vi "Element to Enum Metadata.vi"(8 "error in (no error)":errorcluster, 9 "Name":string, 10 "MessageElementType":T2, 11 "Element":variant) -> (0 "error out":errorcluster, 2 "Is Enum?":bool, 3 "Enum Metadata":T1)   [LabVIEW 2019, in "grpc-lvsupport.lvlib"]
uses:
  grpc-lvsupport.lvlib
  typeDefs/Message Element Type.ctl
  typeDefs/Enum Metadata.ctl
  <vilib>/Utility/Data Type/NI_Data Type.lvlib
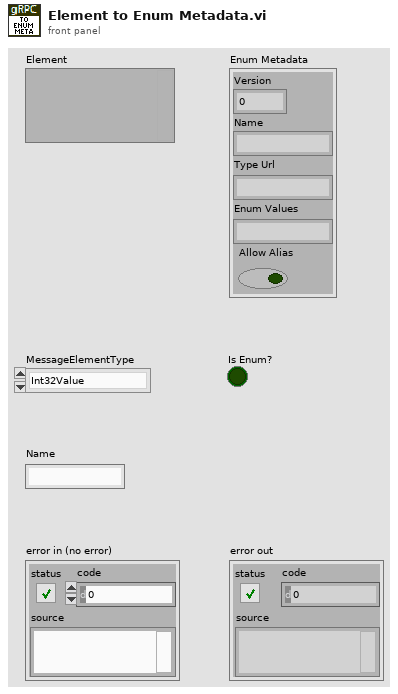
[diagram p1: front panel]
types:
  T1 = typedef "grpc-lvsupport.lvlib/Enum Metadata.ctl" = cluster{"Version":i32, "Name":string, "Type Url":string, "Enum Values":string, "Allow Alias":bool}
  T2 = typedef "grpc-lvsupport.lvlib/Message Element Type.ctl" = enum32{"Int32Value", "FloatValue", "DoubleValue", "BoolValue", "StringValue", "MessageValue", "Int64Value", "UInt32Value", "UInt64Value", "EnumValue", "Bytes", "Fixed64", "Fixed32", "SFixed64", "SFixed32", "SInt64", "SInt32"}
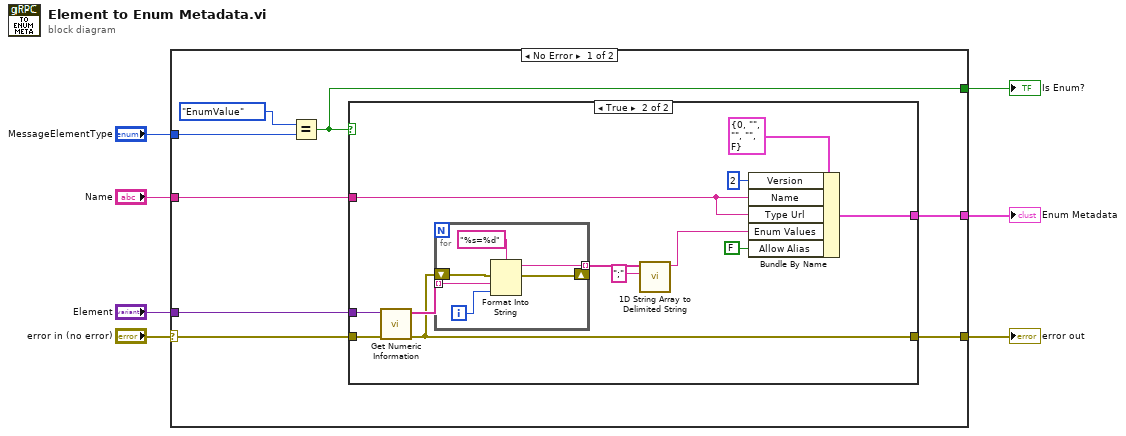
[diagram p0: block diagram]
diagram:
  n1 = case shown="No Error" "error in (no error)" {
    selector: "error in (no error)" -> [w11 w35]
    tunnel: "MessageElementType" -> [w15 _]
    tunnel: [w13 w35] -> w5
    tunnel: "Element" -> [w12 _]
    tunnel: [w10 _] -> w3
    tunnel: [w9 _] -> w2
    tunnel: "Name" -> [w8 _]
    frame No Error {
      n2 = Equal?(x=Message_Element_Type."EnumValue", y=w15) -> (x = y?=w10:bool)
      n3 = case shown="True" w10 {
        tunnel: [w16 w22] -> w13
        tunnel: w12 -> [_ w28]
        tunnel: w11 -> [w16 w27]
        tunnel: [_ w18] -> w9
        tunnel: w8 -> [_ w17]
        frame False {
        }
        frame True {
          n4 = call <vilib>:"Get Numeric Information.vi"("error in (no error)"=w27, "variant"=w28) -> ("error out"=w22:errorcluster, "enum names"=w23:string[])  [unwired: 6 in, 2 out]
          n5 = for {
            tunnel: w23 -> [w34] mode=indexing
            shift-right: [w30] -> _
            shift-left: w22 -> [w31]
            tunnel: [w29] -> w21 mode=indexing
            i -> [w33]
            n6 = Format Into String(format string="%s=%d", error in=w31, w34, w33) -> (resulting string=w29:string, error out=w30:errorcluster)  [unwired: 1 in]
          }
          n7 = call <vilib>:"1D String Array to Delimited String.vi"("delimiter"=";", "string array"=w21) -> ("delimited string"=w19:string)  [unwired: 9 in]
          n8 = Bundle By Name(cluster=T1 {"Version"=0, "Name"="", "Type Url"="", "Enum Values"="", "Allow Alias"=FALSE} ("Enum Metadata"), "Version"=2, "Name"=w17, "Type Url"=w17, "Enum Values"=w19, "Allow Alias"=FALSE) -> (w18:T1)
        }
      }
    }
    frame Error {
    }
  }
  "error out" <- w5
  "Is Enum?" <- w3
  "Enum Metadata" <- w2
